vi "Execute.vi"(8 "Error In":errorcluster, 11 "Display Manager In":refnum<class "Display Manager.lvclass">) -> (0 "Error Out":errorcluster, 3 "Display Manager Out":refnum<class "Display Manager.lvclass">)   [LabVIEW 2019, in "Display Manager.lvclass"]
uses:
  Display Manager.lvclass
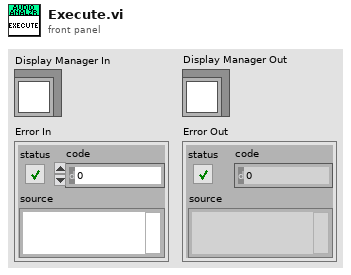
[diagram p1: front panel]
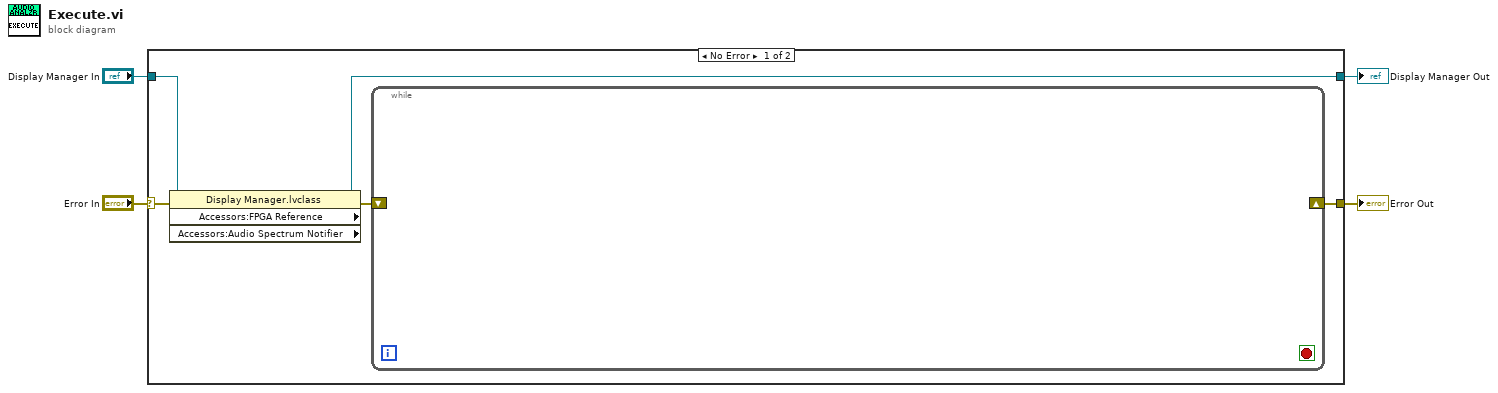
[diagram p0: block diagram]
diagram:
  n1 = case shown="No Error" "Error In" {
    selector: "Error In" -> [w8 w11]
    tunnel: [w9 w11] -> w3
    tunnel: "Display Manager In" -> [w7 w10]
    tunnel: [w5 w10] -> w1
    frame No Error {
      n2 = property class="Display Manager.lvclass" props=["Accessors:FPGA Reference", "Accessors:Audio Spectrum Notifier"](reference=w7, error in=w8) -> (reference out=w5:refnum<class "Display Manager.lvclass">, error out=w6:errorcluster)  [unwired: 2 out]
      n3 = while {
        shift-right: [_] -> w9
        shift-left: w6 -> [_]
        stop <- _ stop-if-true
      }
    }
    frame Error {
    }
  }
  "Error Out" <- w3
  "Display Manager Out" <- w1
